vi "Show.vi"(6 "timeout in ms (-1)":i32=-1, 8 "error in (no error)":errorcluster, 11 "module in":refnum<class "UIManager.lvclass">) -> (0 "error out":errorcluster, 3 "module out":refnum<class "UIManager.lvclass">, 4 "timed out?":bool)   [LabVIEW 2024, in "UIManager.lvclass"]
uses:
  UIManager.lvclass
  C:/DevOps/CORTEX/JQMH/JQMHCore/Module/RQMHModule.lvclass
  JQMHCore/Module/Reply.ctl
  UIManager.lvclass/UIManager.ctl
  Show ReplyArgs.ctl
  Show Args.ctl
  JQMHCore/Module/RQMHModule.lvclass
  C:/DevOps/CORTEX/JQMH/ModuleTemplates/UIManager/UIManager.lvclass
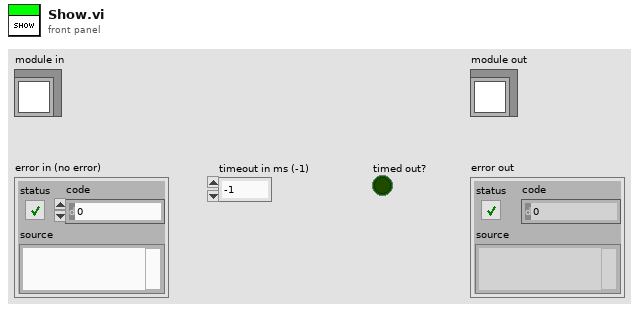
[diagram p1: front panel]
types:
  T1 = typedef "UIManager.lvclass/Show Args.ctl" = cluster{"String":string}
  T2 = typedef "RQMHModule.lvclass/Reply.ctl" = cluster{"Expects Reply":bool, "Reply":refnum<notifier>}
  T3 = typedef "UIManager.lvclass/Show ReplyArgs.ctl" = cluster{"Boolean":bool}
  T4 = cluster{"RQMH_REPLYARGS":T3, "error in (no error)":errorcluster}
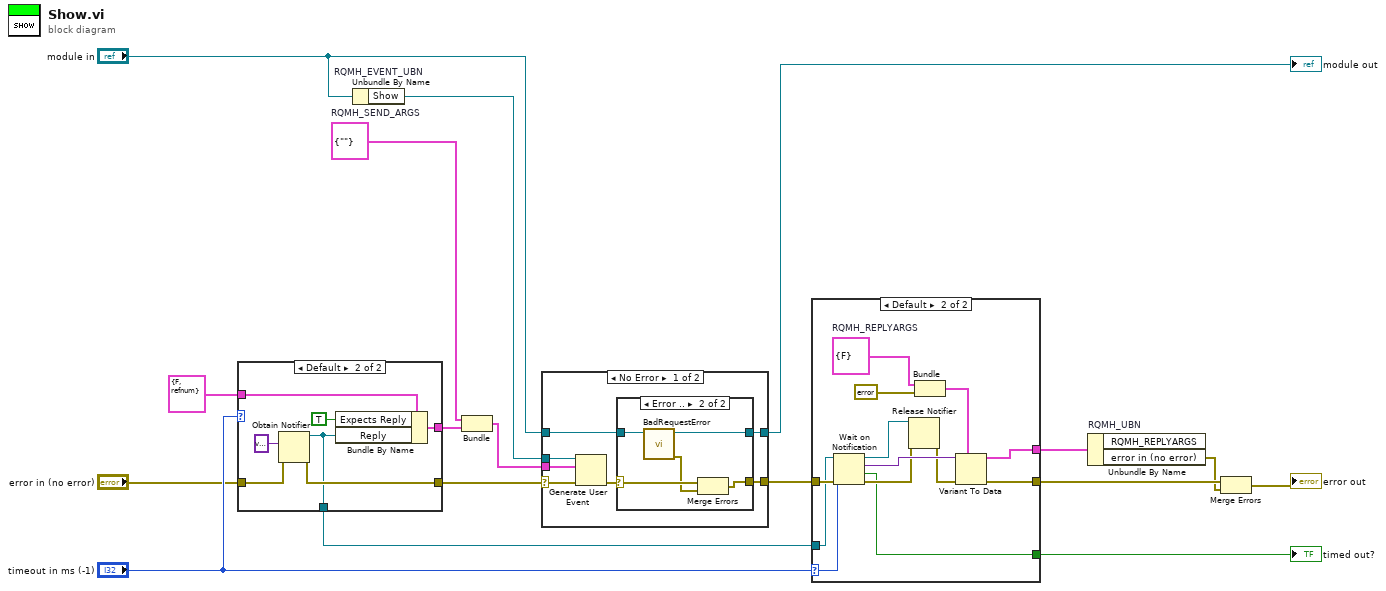
[diagram p0: block diagram]
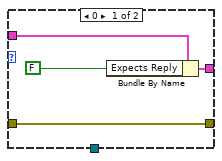
[diagram p4: hidden frame]
diagram:
  w5 = T1 {"String"=""}  # RQMH_SEND_ARGS
  n1 = case shown="Default" "timeout in ms (-1)" {
    tunnel: [w20 w27] -> w17
    tunnel: "error in (no error)" -> [w18 w26]
    tunnel: [w18 w25] -> w15
    tunnel: [_ w24] -> w13
    tunnel: T2 {"Expects Reply"=FALSE, "Reply"=refnum} ("Reply") -> [w21 w23]
    frame 0 {
      n2 = Bundle By Name(cluster=w21, "Expects Reply"=FALSE) -> (w20:T2)
    }
    frame Default {
      n3 = Obtain Notifier(notification data type=variant, error in (no error)=w26) -> (notifier out=w24:refnum<notifier>, error out=w25:errorcluster)  [unwired: 2 in, 1 out]
      n4 = Bundle By Name(cluster=w23, "Expects Reply"=TRUE, "Reply"=w24) -> (w27:T2)
    }
  }
  n5 = Unbundle By Name "RQMH_EVENT_UBN"("module in") -> ("Show"=w6:refnum<user-event>)
  n6 = Bundle("RQMH_SEND_ARGS"=w5, "Reply"=w17) -> (w16:cluster{"RQMH_SEND_ARGS":T1, "Reply":T2})  [unwired: 1 in]
  n7 = case shown="No Error" w15 {
    selector: w15 -> [w32 w43]
    tunnel: w16 -> [w35 _]
    tunnel: w6 -> [w34 _]
    tunnel: [w31 w43] -> w14
    tunnel: "module in" -> [w30 w44]
    tunnel: [w29 w44] -> w8
    frame No Error {
      n8 = Generate User Event(user event=w34, event data cluster=w35, error in=w32) -> (error out=w33:errorcluster)  [unwired: 1 in, 1 out]
      n9 = case shown="Error .." w33 {
        selector: w33 -> [w36 w42]
        tunnel: [w36 w41] -> w31
        tunnel: w30 -> [w37 w40]
        tunnel: [w37 w39] -> w29
        frame No Error {
        }
        frame Error {
          n10 = call "BadRequestError.vi"("JQMHModule in"=w40) -> ("error out"=w38:errorcluster, "JQMHModule out"=w39:refnum<class "UIManager.lvclass">)  [unwired: 9 in]
          n11 = Merge Errors(w42, w38) -> (w41:errorcluster)
        }
      }
    }
    frame Error {
    }
  }
  "module out" <- w8
  n12 = case shown="Default" "timeout in ms (-1)" {
    selector: "timeout in ms (-1)" -> [_ w49]
    tunnel: w14 -> [w45 w58]
    tunnel: w13 -> [_ w57]
    tunnel: [_ w50] -> w12
    tunnel: [w45 w47] -> w4
    tunnel: [_ w46] -> w3
    frame 0 {
    }
    frame Default {
      w48 = T3 {"Boolean"=FALSE}  # RQMH_REPLYARGS
      n13 = Wait on Notification(notifier=w57, timeout in ms (-1)=w49, error in (no error)=w58) -> (notifier out=w53:refnum<notifier>, notification=w54:variant, timed out?=w50:bool, error out=w52:errorcluster)  [unwired: 1 in]
      n14 = Release Notifier(notifier=w53, error in (no error)=w52) -> (error out=w51:errorcluster)  [unwired: 1 in, 2 out]
      n15 = Bundle("RQMH_REPLYARGS"=w48, "error in (no error)"=errorcluster {"status"=FALSE, "code"=0, "source"=""}) -> (w56:T4)  [unwired: 1 in]
      n16 = Variant To Data(error in=w51, type=w56, Variant=w54) -> (data=w46:T4, error out=w47:errorcluster)
    }
  }
  "timed out?" <- w12
  n17 = Unbundle By Name "RQMH_UBN"(w3) -> ("error in (no error)"=w1:errorcluster)  [unwired: 1 out]
  n18 = Merge Errors(w4, w1) -> (→"error out":errorcluster)
